vi "Call First SubVI Async.vi"(11 "logger in":refnum<class "Logger.lvclass">) -> (3 "logger out":refnum<class "Logger.lvclass">)   [LabVIEW 2018]
uses:
  src/api/logger_class/Logger.lvclass
  src/api/logger_class/Log Levels.ctl
  src/api/logger_class/Log (Parts).vi
  First SubVI.vi
  Scope Tester Class.lvclass
panel:
  # "Connector Pane"
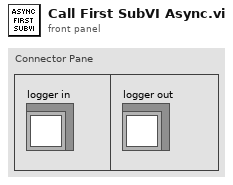
[diagram p1: front panel]
types:
  T1 = typedef "GLog.lvlib/Logger.lvclass/Log Levels.ctl" = enum16{"Trace", "Debug", "Info", "Warning", "Error", "Critical"}
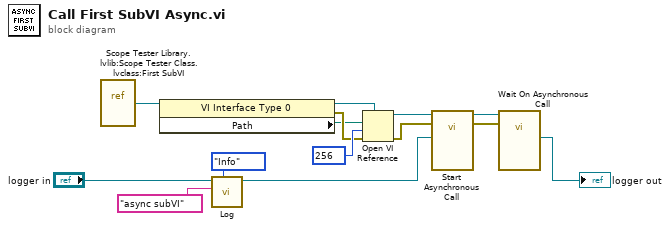
[diagram p0: block diagram]
diagram:
  n1 = vi-ref "Scope Tester Library.lvlib:Scope Tester Class.lvclass:First SubVI.vi"() -> (w6:refnum<vi>)
  n2 = property class="VI Interface Type 0"(reference=w6) -> (reference out=w8:refnum<vi>, error out=w11:errorcluster, "Path"=w7:path)  [unwired: 1 in]
  n3 = call-poly "Log.vi"("log level"=Log_Levels."Info" ("level"), "message"="async subVI", "logger in"="logger in") -> ("logger out"=w1:refnum<class "Logger.lvclass">)  [unwired: 8 in]
  n4 = Open VI Reference(type specifier VI Refnum (for type only)=w8, vi path=w7, options=256, error in (no error)=w11) -> (vi reference=w9:refnum<vi>, error out=w10:errorcluster)  [unwired: 2 in]
  n5 = call-by-ref "Start Asynchronous Call"(reference=w9, error in=w10, "logger in"=w1) -> (reference out=w13:refnum<vi>, error out=w14:errorcluster)  [unwired: 10 in, 1 out]
  n6 = call-by-ref "Wait On Asynchronous Call"(reference=w13, error in=w14) -> ("logger out"=→"logger out":refnum<class "Logger.lvclass">)  [unwired: 11 in, 2 out]
